vi "format_http_return_headers.vi"(10 "headers in":string) -> (1 "msg":string, 2 "status code":string, 4 "headers array":string[](array[string]))   [LabVIEW 2018]
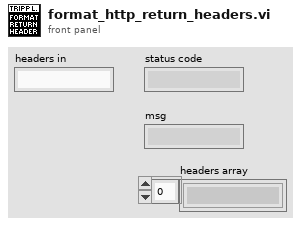
[diagram p1: front panel]
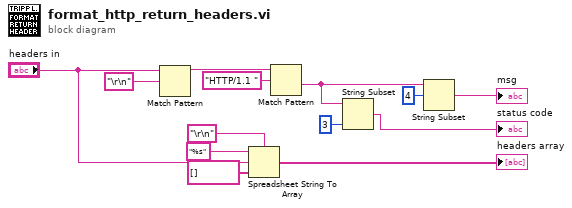
[diagram p0: block diagram]
diagram:
  n1 = Match Pattern(string="headers in", regular expression="\r\n" ("delimiter (Tab)")) -> (before substring=w9:string)  [unwired: 1 in, 3 out]
  n2 = Spreadsheet String To Array(delimiter (Tab)="\r\n", format string="%s", spreadsheet string="headers in", array type (2D Dbl)=string[] []) -> (array=→"headers array":string[])
  n3 = Match Pattern(string=w9, regular expression="HTTP/1.1 ") -> (after substring=w12:string)  [unwired: 1 in, 3 out]
  n4 = String Subset(string=w12, length (rest)=3 ("length (rest)")) -> (substring=→"status code":string)  [unwired: 1 in]
  n5 = String Subset(string=w12, offset (0)=4) -> (substring=→"msg":string)  [unwired: 1 in]
